vi "Write Microscope.vi"(8 "error in (no error)":errorcluster, 10 "Actor Framework:Message Enqueuer":refnum<class "Message Enqueuer.lvclass">, 11 "Virtual Microscope in":refnum<class "Virtual Microscope.lvclass">) -> (0 "error out":errorcluster, 3 "Virtual Microscope out":refnum<class "Virtual Microscope.lvclass">)   [LabVIEW 2015, in "Virtual Microscope.lvlib" / "Virtual Microscope.lvclass"]
uses:
  Virtual Microscope.lvclass
  <vilib>/ActorFramework/Message Enqueuer/Message Enqueuer.lvclass
  Virtual Microscope.lvclass/Virtual Microscope.ctl
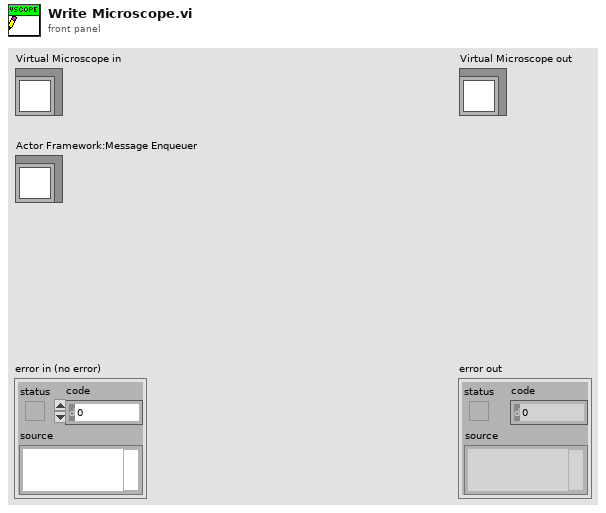
[diagram p1: front panel]
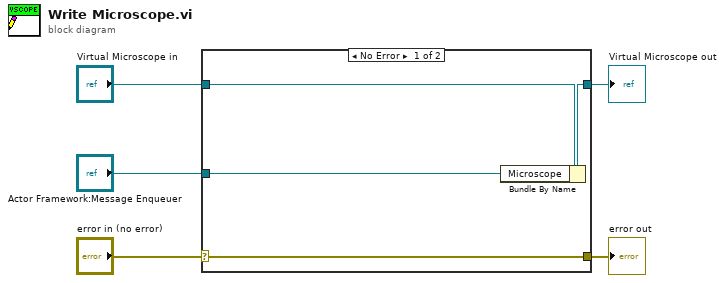
[diagram p0: block diagram]
diagram:
  n1 = case shown="No Error" "error in (no error)" {
    selector: "error in (no error)" -> [w9 w10]
    tunnel: [w9 w10] -> w4
    tunnel: [w7 w11] -> w2
    tunnel: "Virtual Microscope in" -> [w8 w11]
    tunnel: "Actor Framework:Message Enqueuer" -> [w6 _]
    frame No Error {
      n2 = Bundle By Name(cluster=w8, "Microscope"=w6) -> (w7:refnum<class "Virtual Microscope.lvclass">)
    }
    frame Error {
    }
  }
  "error out" <- w4
  "Virtual Microscope out" <- w2
